vi "Config_DC_V.vi"(0 "reference in":refnum<class "DMM_Keysight_34980A.lvclass">, 5 "Range (5:Auto)":T1(ring)=enum."Auto", 7 "Resolution (5:Default)":T2(ring)=enum."Default", 11 "error in (no error)":errorcluster) -> (4 "reference in":refnum<class "DMM_Keysight_34980A.lvclass">, 15 "error out":errorcluster)   [LabVIEW 2022 SP3, in "DMM_Keysight_34980A.lvlib" / "DMM_Keysight_34980A.lvclass"]
uses:
  DMM_Keysight_34980A.lvclass
  Mode.ctl
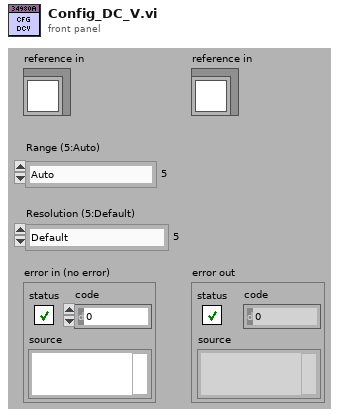
[diagram p1: front panel]
types:
  T1 = enum16{"100 mV", "1 V", "10 V", "100 V", "300 V", "Auto", "Minimum", "Maximum"}
  T2 = enum16{"4 1/2", "5 1/2", "6 1/2", "Least", "Highest", "Default"}
  T3 = typedef "DMM_Keysight_34980A.lvlib/DMM_Keysight_34980A.lvclass/Mode.ctl" = enum16{"DCV", "ACV", "2W Ohms", "4W Ohms", "Frequency", "DCA", "ACA"}
  T4 = typedef "DMM_Keysight_34980A.lvlib/DMM_Keysight_34980A.lvclass/ObjectAttributes.ctl" = cluster{"Config":T5, "VISA ref":refnum<visa-resource-name>, "Meas":dbl, "Range DCV":enum16{"100 mV", "1 V", "10 V", "100 V", "300 V", "Auto", "Minimum", "Maximum"}, "Range ACV":enum16{"100 mV", "1 V", "10 V", "100 V", "300 V", "Auto", "Minimum", "Maximum", "Default"}, "Range Ohms":enum16{"100 Ohm", "1 kOhm", "10 kOhm", "100 kOhm", "1 MOhm", "10 MOhm", "100 MOhm", "Auto", "Minimum", "Maximum"}, "Range VFreq":enum16{"100 mV", "1 V", "10 V", "100 V", "300 V", "Auto", "Minimum", "Maximum"}, " Range ACA":enum16{"10 mA", "100 mA", "1 A", "Auto", "Minimum", "Maximum"}, " Range DCA":enum16{"10 mA", "100 mA", "1 A", "Auto", "Minimum", "Maximum"}, "Mode":T3, "Resolution":enum16{"4 1/2", "5 1/2", "6 1/2", "Least", "Highest", "Default"}, "Bandwidth":enum16{"3 Hz", "20 Hz", "200 Hz", "Minimum", "Maximum"}, "Low Frequency":enum16{"3 Hz", "20 Hz", "200 Hz", "Minimum", "Maximum"}, "Aperture":enum16{"10 ms", "100 ms", "1 sec", "Minimum", "Maximum"}, "Measurement":dbl[], "Time":dbl[], "Samples":u32, "dt":dbl, "Timeout":dbl}
  T5 = typedef "DMM_Keysight_34980A.lvlib/DMM_Keysight_34980A.lvclass/Config.ctl" = cluster{"VISA":refnum<visa-resource-name>}
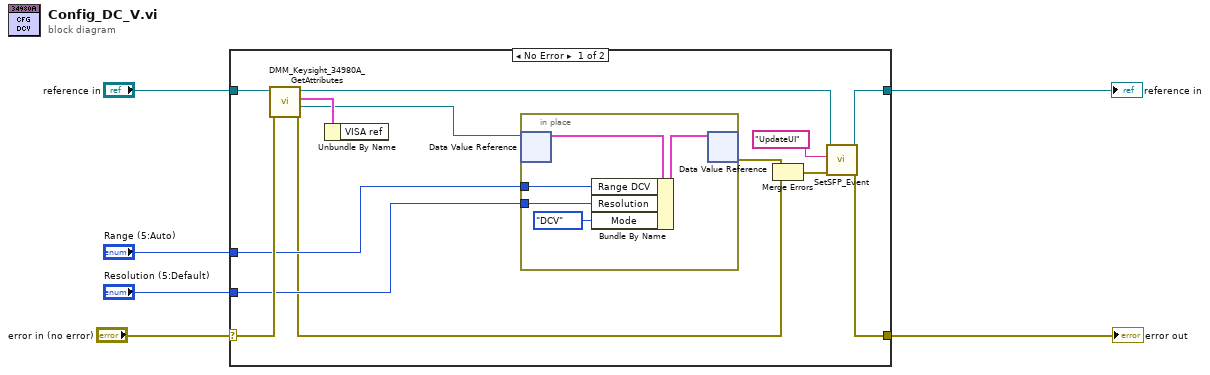
[diagram p0: block diagram]
diagram:
  n1 = case shown="No Error" "error in (no error)" {
    selector: "error in (no error)" -> [w19 w26]
    tunnel: [w10 w26] -> w5
    tunnel: [w11 w25] -> w3
    tunnel: "reference in" -> [w17 w25]
    tunnel: "Resolution (5:Default)" -> [w8 _]
    tunnel: "Range (5:Auto)" -> [w9 _]
    frame No Error {
      n2 = call "DMM_Keysight_34980A_GetAttributes.vi"("error in (no error)"=w19, "reference in"=w17) -> ("error out"=w7:errorcluster, "DataRef"=w13:refnum<data-value>, "Data"=w18:T4, "reference out"=w12:refnum<class "DMM_Keysight_34980A.lvclass">)  [unwired: 6 in]
      n3 = Unbundle By Name(w18) -> ()  [unwired: 1 out]
      n4 = in-place {
        in-place-border: w9 -> [w22]
        in-place-border: w8 -> [w21]
        n5 = in-place-dvr #1(w13) -> (w24:T4)  [unwired: 1 out]
        n6 = Bundle By Name(cluster=w24, "Range DCV"=w22, "Resolution"=w21, "Mode"=Mode."DCV") -> (w23:T4)
        n7 = in-place-dvr #1(w23) -> (w16:errorcluster)  [unwired: 1 out]
      }
      n8 = Merge Errors(w16, w7) -> (w15:errorcluster)
      n9 = call-dynamic "SetSFP_Event.vi"("error in (no error)"=w15, "msg"="UpdateUI", "reference in"=w12) -> ("error out"=w10:errorcluster, "reference out"=w11:refnum<class "DMM_Keysight_34980A.lvclass">)  [unwired: 7 in]
    }
    frame Error {
    }
  }
  "error out" <- w5
  "reference in" <- w3
